vi "test-timer.vi"() -> ()   [LabVIEW 2019]
uses:
  <vilib>/Rock Robotics/WPI/ThirdParty/JAS_Junk/TrajLib/TIMER.ctl
  <vilib>/Rock Robotics/WPI/ThirdParty/JAS_Junk/TrajLib/Trajectory_Library.lvlib
panel:
  in  "STOP":bool
  out "Done":bool
  in  "Period":dbl
  in  "GO":bool
  out "CurrentTImer 2":dbl
  out "CurrentTImer":dbl
  out "TIMER 2":T1 {"Accumulated TIme" format="%13.5p"; "StartTime" format="%13.5p"}
  out "TIMER":T1 {"Accumulated TIme" format="%13.5p"; "StartTime" format="%13.5p"}
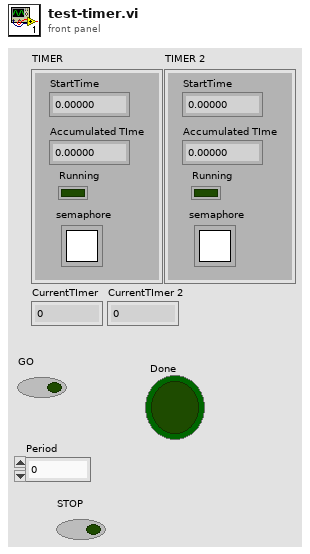
[diagram p1: front panel]
types:
  T1 = typedef "Trajectory_Library.lvlib/TIMER.ctl" = cluster{"StartTime":dbl, "Accumulated TIme":dbl, "Running":bool, "semaphore":T2}
  T2 = typedef "Semaphore RefNum" = refnum<k1>
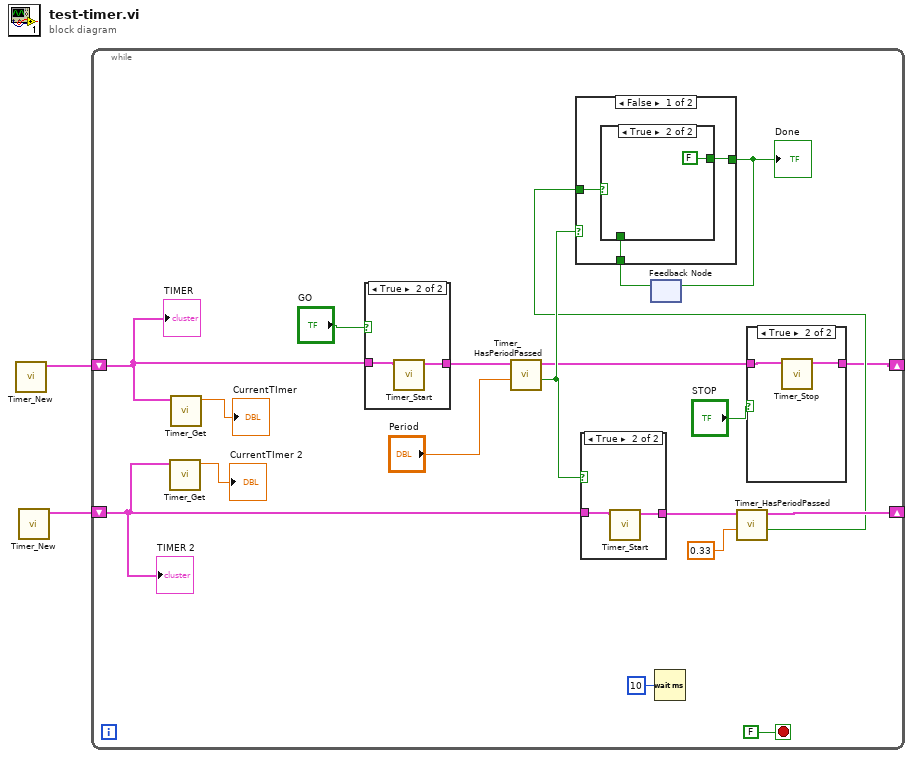
[diagram p0: block diagram]
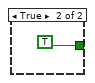
[diagram p4: hidden frame]
diagram:
  n1 = call <vilib>:"Timer_New.vi"() -> ("TIMER"=w1:T1)  [unwired: 11 in]
  n2 = call <vilib>:"Timer_New.vi"() -> ("TIMER"=w2:T1)  [unwired: 11 in]
  n3 = while {
    shift-right: [w3] -> _
    shift-left: w1 -> [w16]
    shift-right: [w8] -> _
    shift-left: w2 -> [w13]
    stop <- FALSE stop-if-true
    n4 = call <vilib>:"Timer_Get.vi"("TIMER"=w13) -> ("CurrentTImer"=→"CurrentTImer 2":dbl)  [unwired: 10 in]
    n5 = call <vilib>:"Timer_Get.vi"("TIMER"=w16) -> ("CurrentTImer"=→"CurrentTImer":dbl)  [unwired: 10 in]
    n6 = case shown="True" "GO" {
      tunnel: w16 -> [w34 w36]
      tunnel: [w34 w35] -> w15
      frame False {
      }
      frame True {
        n7 = call <vilib>:"Timer_Start.vi"("in Timer"=w36) -> ("out Timer"=w35:T1)  [unwired: 10 in]
      }
    }
    n8 = call <vilib>:"Timer_HasPeriodPassed.vi"("Period"="Period", "in Timer"=w15) -> ("Expired"=w12:bool, "out Timer"=w4:T1)  [unwired: 7 in, 1 out]
    n9 = case shown="True" w12 {
      tunnel: w13 -> [w31 w33]
      tunnel: [w31 w32] -> w9
      frame False {
      }
      frame True {
        n10 = call <vilib>:"Timer_Start.vi"("in Timer"=w33) -> ("out Timer"=w32:T1)  [unwired: 10 in]
      }
    }
    n11 = feedback #1() -> (w10:bool)  [unwired: 1 in]
    n12 = Wait (ms)(milliseconds to wait=u32 10) -> ()  [unwired: 1 out]
    n13 = call <vilib>:"Timer_HasPeriodPassed.vi"("Period"=0.33, "in Timer"=w9) -> ("Expired"=w7:bool, "out Timer"=w8:T1)  [unwired: 7 in, 1 out]
    n14 = case shown="False" w12 {
      tunnel: [w27 TRUE] -> w11
      tunnel: w10 -> [w26 _]
      tunnel: w7 -> [w25 _]
      frame False {
        n15 = case shown="True" w25 {
          tunnel: [w28 FALSE] -> w27
          tunnel: w26 -> [w28 _]
          frame False {
          }
          frame True {
          }
        }
      }
      frame True {
      }
    }
    "Done" <- w11
    n16 = feedback-in #1(w11) -> ()
    n17 = case shown="True" "STOP" {
      tunnel: w4 -> [w22 w23]
      tunnel: [w22 w24] -> w3
      frame False {
      }
      frame True {
        n18 = call <vilib>:"Timer_Stop.vi"("in Timer"=w23) -> ("out Timer"=w24:T1)  [unwired: 10 in]
      }
    }
    "TIMER" <- w16
    "TIMER 2" <- w13
  }
